vi "PE7265Monitor.vi"(0 "Lock-in Reference":u16(ring) items=["Lock-in 1", "Lock-in 2", "Lock-in 3"]) -> ()   [LabVIEW 2019]
uses:
  Utility/Monitor Communication/PE7265/PE7265-Cluster.ctl
  Utility/PE7260/PE7625-Settings.ctl
  Instrument_Setup.vi
  Global/Global Variables/Data_Display_global.vi
panel:
  out "PE7625-Settings":T1={"PE7265 AutoSens at ech step"=FALSE, "PE7265 Sens"=26, "Coupling"=FALSE, "AC Gain"=3, "Auto AC Gain"=FALSE, "Input Device (Voltage Mode)"=TRUE, "Line Frequency"=TRUE, "Input Connector Shells"=FALSE, "PE7265 Input Mode"=3, "Line Frequency\nRejection Filter"=1, "Port"=0, "7265 GPIB Address"=12, "Interface"=FALSE, "Exit"=FALSE, "GPIB Parameter 7260"={"address"="12", "delay time"=10.0, "mode"=6}, "PE7265 delay after AS"=10.0, "VISA session PE7265"="GPIB0::12::INSTR", "Slope"=1, "Synchronous TC"=TRUE, "Time Constant"=15, "Reference I/P"=0, "Reference\nHarmonic"=1, "Oscillator Amplitude (Volts rms)"=1.5, "Oscillator Frequency (Hz)"=19.0, "Ref Unlocked"=FALSE, "Virtual Reference\nMode"=FALSE} {"Oscillator Frequency (Hz)" min=0.001 max=250000.0 step=0.001 format="%.3f"; "Oscillator Amplitude (Volts rms)" min=0.0 max=5.0 step=1e-06 format="%.6f"; "Reference\nHarmonic" min=1 step=1; "Reference I/P" items=["Internal", "External TTL (Rear Panel)", "External (Front Panel)"]; "Time Constant" items=["10µs", "20µs", "40µs", "80µs", "160µs", "320µs", "640µs", "5ms", "10ms", "20ms", "50ms", "100ms", "200ms", "500ms", "1s", "2s", "5s", "10s", "20s", "50s", "100s", "200s", "500s", "1ks", "2ks", "5ks", "10ks", "20ks", "50ks", "100ks"]; "Slope" items=["6db/octave", "12dB/octave", "18dB/octave", "24dB/octave"]; "PE7265 delay after AS" format="%.2f"; "GPIB Parameter 7260"."delay time" format="%.2f"; "7265 GPIB Address" min=1 max=32 step=1; "Port" items=["COM 1", "COM 2", "COM 3", "COM 4", "COM 5", "COM 6", "COM 7", "COM 8", "COM 9", "COM 10"]; "Line Frequency\nRejection Filter" items=["OFF", "F", "2F", "F & 2F"]; "PE7265 Input Mode" items=["Inputs Grounded (test)", "A (Single-Ended Voltage)", "-B (Inverting Single Ended Voltage)", "A-B (Differential Voltage)", "B Current input - High Bandwidth", "B Current input - Low Noise"]; "AC Gain" items=["0dB", "10dB", "20dB", "30dB", "40dB", "50dB", "60dB", "70dB", "80dB", "90dB"]; "PE7265 Sens" items=["2nV", "5nV", "10nV", "20nV", "50nV", "100nV", "200nV", "500nV", "1µV", "2µV", "5µV", "10µV", "20µV", "50µV", "100µV", "200µV", "500µV", "1mV", "2mV", "5mV", "10mV", "20mV", "50mV", "100mV", "200mV", "500mV", "1V"]}
  out "Sensitivity 2":i16(ring)=15 items=["2 nV", "5 nV", "10 nV", "20 nV", "50 nV", "100 nV", "200 nV", "500 nV", "1 µV", "2 µV", "5 µV", "10 µV", "20 µV", "50 µV", "100 µV", "200 µV", "500 µV", "1 mV", "2 mV", "5 mV", "10 mV", "20 mV", "50 mV", "100 mV", "200 mV", "500 mV", "1 V", ""]
  in  "Stopp":bool
  out "PE7265-Cluster":T2={"Lockin 1"=[], "X1-Display"=0.0, "X1 Percent"=0.0, "Y1-Display"=0.0, "X1 Percent 2"=0.0, "Unit X1"="nV", "Unit X1a"="nV", "Unit X2"="nV", "Unit X2a"="nV", "X1 Overload"=FALSE, "Y1 Overload"=FALSE, "Sensitivity Setpoint"=26, "X1"=0.0, "Y1"=0.0} {"Sensitivity Setpoint" items=["2 nV", "5 nV", "10 nV", "20 nV", "50 nV", "100 nV", "200 nV", "500 nV", "1 µV", "2 µV", "5 µV", "10 µV", "20 µV", "50 µV", "100 µV", "200 µV", "500 µV", "1 mV", "2 mV", "5 mV", "10 mV", "20 mV", "50 mV", "100 mV", "200 mV", "500 mV", "1 V", ""]; "X1 Percent 2" scale=0.0..1.0; "X1 Percent" scale=0.0..1.0; "X1-Display" format="%#4_5f"}
  # "Input Configuration"
  # "RS232"
  # "GPIB"
  # "Uses VISA Communications"
  # "Sensitivity"
  # "Float"
  # "50 Hz"
  # "DC"
  # "Ground"
  # "60 Hz"
  # "AC"
  # "Bipolar - Input Impedance 10 k"
  # "On"
  # "FET - Input Impedance 10 M"
  # "Off"
  # "Output Channels"
  # "Reference Channel - Single Reference"
  # "On"
  # "Off"
  # "On"
  # "Off"
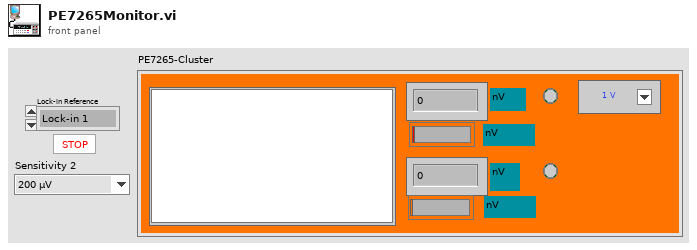
[diagram p1: front panel]
types:
  T1 = typedef "PE7625-Settings.ctl" = cluster{"PE7265 AutoSens at ech step":bool, "PE7265 Sens":i32, "Coupling":bool, "AC Gain":u16, "Auto AC Gain":bool, "Input Device (Voltage Mode)":bool, "Line Frequency":bool, "Input Connector Shells":bool, "PE7265 Input Mode":u16, "Line Frequency\nRejection Filter":u8, "Port":u16, "7265 GPIB Address":i8, "Interface":bool, "Exit":bool, "GPIB Parameter 7260":cluster{"address":string, "delay time":dbl, "mode":i32}, "PE7265 delay after AS":dbl, "VISA session PE7265":refnum<visa-resource-name>, "Slope":u8, "Synchronous TC":bool, "Time Constant":u16, "Reference I/P":u8, "Reference\nHarmonic":u16, "Oscillator Amplitude (Volts rms)":dbl, "Oscillator Frequency (Hz)":dbl, "Ref Unlocked":bool, "Virtual Reference\nMode":bool}
  T2 = typedef "PE7265-Cluster.ctl" = cluster{"Lockin 1":dbl[][], "X1-Display":dbl, "X1 Percent":dbl, "Y1-Display":dbl, "X1 Percent 2":dbl, "Unit X1":string, "Unit X1a":string, "Unit X2":string, "Unit X2a":string, "X1 Overload":bool, "Y1 Overload":bool, "Sensitivity Setpoint":i16, "X1":dbl, "Y1":dbl}
  T3 = cluster{"PE7265 AutoSens at ech step":bool, "PE7265 Sens":i32, "Coupling":bool, "AC Gain":u16, "Auto AC Gain":bool, "Input Device (Voltage Mode)":bool, "Line Frequency":bool, "Input Connector Shells":bool, "PE7265 Input Mode":u16, "Line Frequency\nRejection Filter":u8, "Port":u16, "7265 GPIB Address":i8, "Interface":bool, "Exit":bool, "GPIB Parameter 7260":cluster{"address":string, "delay time":dbl, "mode":i32}, "PE7265 delay after AS":dbl, "VISA session PE7265":refnum<visa-resource-name>, "Slope":u8, "Synchronous TC":bool, "Time Constant":u16, "Reference I/P":u8, "Reference\nHarmonic":u16, "Oscillator Amplitude (Volts rms)":dbl, "Oscillator Frequency (Hz)":dbl, "Ref Unlocked":bool, "Virtual Reference\nMode":bool}
  T4 = cluster{"address":string, "delay time":dbl, "mode":i32}
  T5 = cluster{"Sensitivity Setpoint 1":i32, "Sensitivity Setpoint 2":i32, "Sensitivity Setpoint 3":i32}
  T6 = cluster{"LIA7230-Running":bool, "LIA7230-Running 2":bool, "LIA7230-Running 3":bool, "SR830-Running":bool, "SR830-Running 2":bool, "SR830-Running 3":bool, "PE7265-running":bool, "zurich_Lock_in-running":bool}
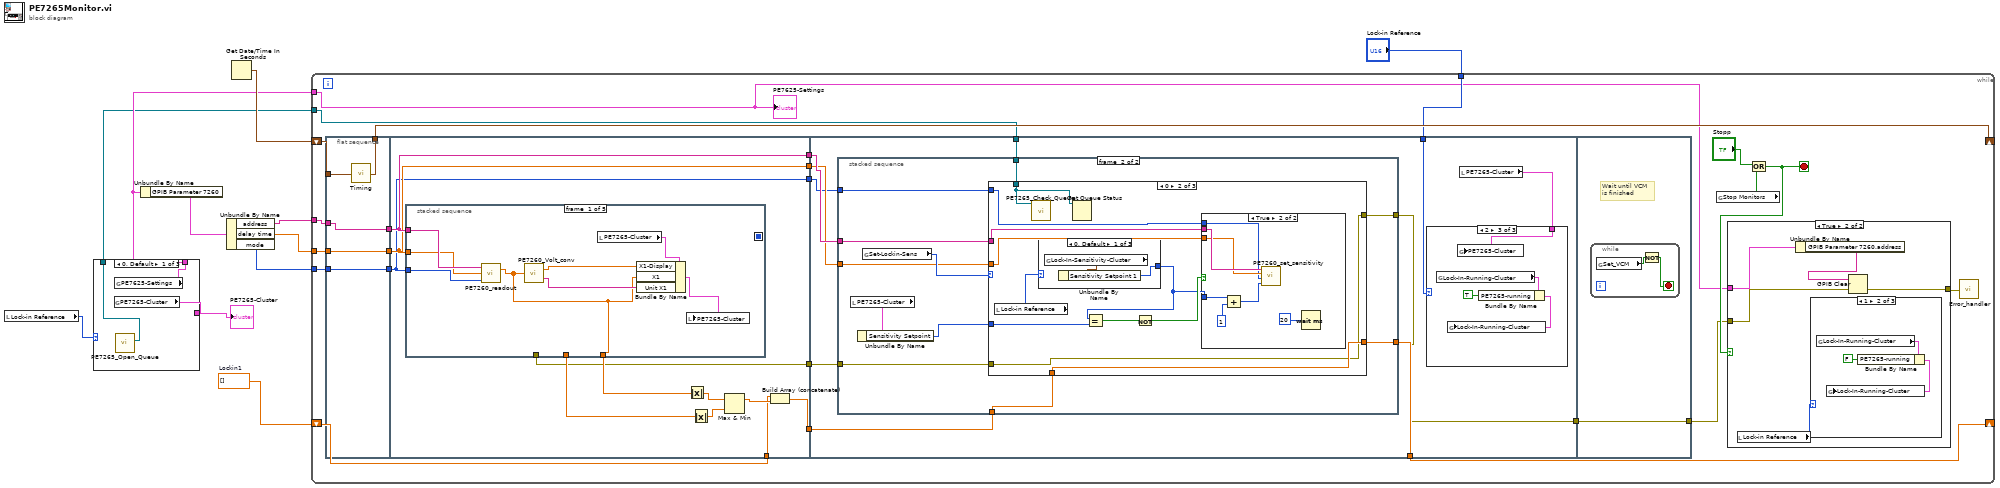
[diagram p0: block diagram]
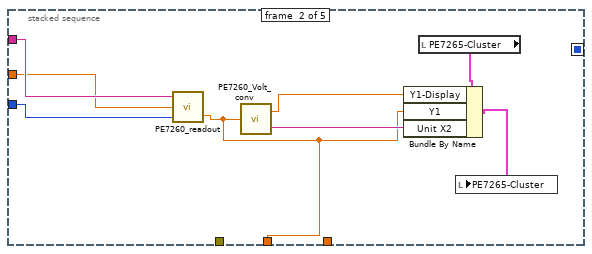
[diagram p2: hidden frame]
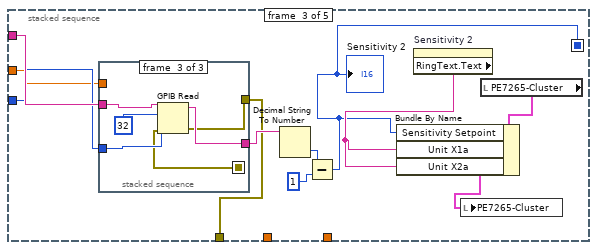
[diagram p3: hidden frame]
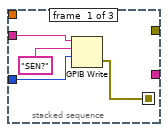
[diagram p4: hidden frame]
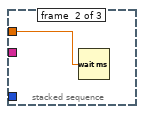
[diagram p5: hidden frame]
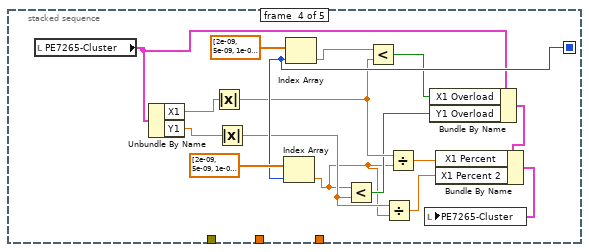
[diagram p6: hidden frame]
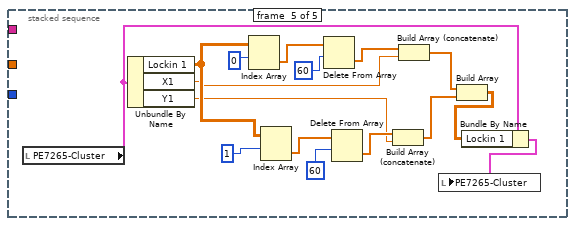
[diagram p7: hidden frame]
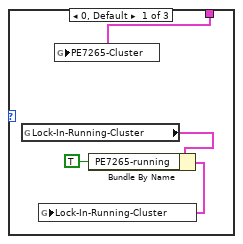
[diagram p8: hidden frame]
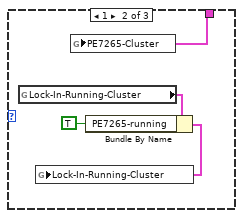
[diagram p9: hidden frame]
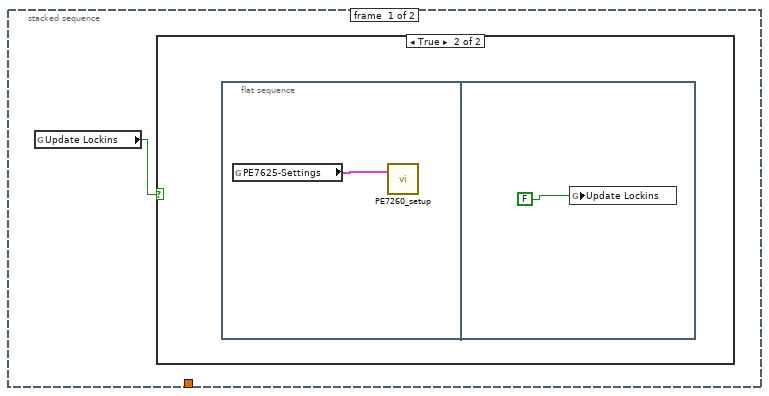
[diagram p10: hidden frame]
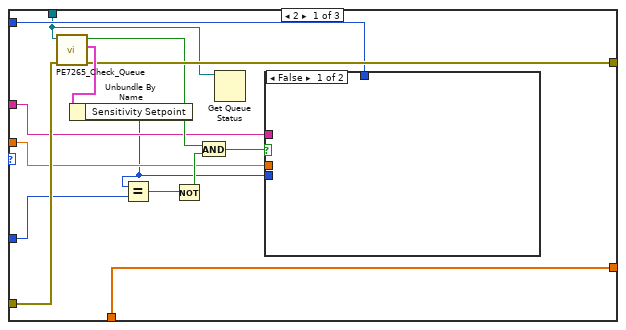
[diagram p12: hidden frame]
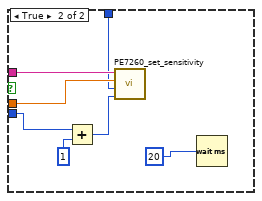
[diagram p13: hidden frame]
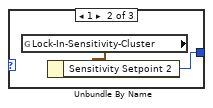
[diagram p15: hidden frame]
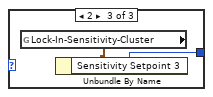
[diagram p16: hidden frame]
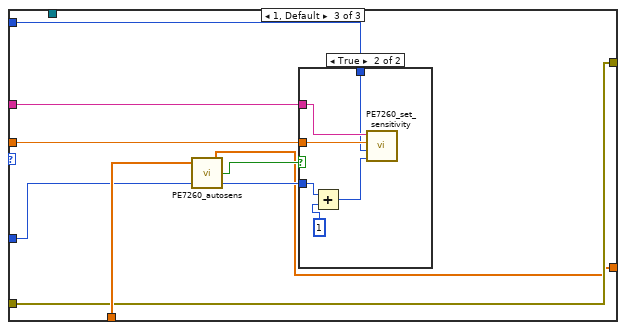
[diagram p17: hidden frame]
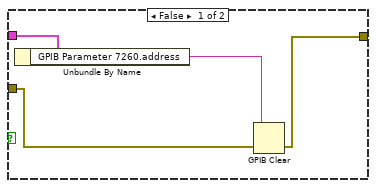
[diagram p19: hidden frame]
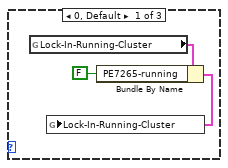
[diagram p20: hidden frame]
diagram:
  w4 = dbl[] []  # Lockin1
  n1 = local read "Lock-in Reference"() -> (w11:u16)
  n2 = case shown="0, Default" w11 {
    tunnel: [w14 w17 w20] -> w7
    tunnel: [w13 w16 w19] -> w10
    tunnel: [w12 w15 w18] -> w3
    frame 0, Default {
      n3 = global read "Data_Display_global.vi" "PE7265-Cluster"() -> (w13:T2)
      n4 = global read "Instrument_Setup.vi" "PE7625-Settings"() -> (w14:T3)
      n5 = call "PE7265_Open_Queue.vi"() -> ("queue out"=w12:refnum<queue>)  [unwired: 10 in, 1 out]
    }
    frame 2 {
      n6 = global read "Instrument_Setup.vi" "PE7625-Settings"() -> (w17:T3)
      n7 = global read "Data_Display_global.vi" "PE7265-Cluster"() -> (w16:T2)
      n8 = call "PE7265_Open_Queue.vi"() -> ("queue out"=w15:refnum<queue>)  [unwired: 10 in, 1 out]
    }
    frame 1 {
      n9 = global read "Instrument_Setup.vi" "PE7625-Settings"() -> (w20:T3)
      n10 = global read "Data_Display_global.vi" "PE7265-Cluster"() -> (w19:T2)
      n11 = call "PE7265_Open_Queue.vi"() -> ("queue out"=w18:refnum<queue>)  [unwired: 10 in, 1 out]
    }
  }
  "PE7265-Cluster" <- w10
  n12 = Unbundle By Name(w7) -> ("GPIB Parameter 7260"=w9:T4)
  n13 = Unbundle By Name(w9) -> ("address"=w1:string, "delay time"=w6:dbl, "mode"=w5:i32)
  n14 = Get Date/Time In Seconds() -> (seconds since 1Jan1904=w8:timestamp)
  n15 = while {
    tunnel: w1 -> [w39]
    shift-right: [w40] -> _
    shift-left: w8 -> [w41]
    tunnel: w7 -> [w21]
    tunnel: w6 -> [w37]
    tunnel: w5 -> [w35]
    shift-right: [w25] -> _
    shift-left: w4 -> [w33]
    tunnel: w3 -> [w24]
    tunnel: "Lock-in Reference" -> [w23]
    stop <- w27 stop-if-true
    n16 = flat-sequence {
      tunnel: w41 -> [w49]
      tunnel: [w48] -> w40
      tunnel: w39 -> [w47]
      tunnel: [w47] -> w38
      tunnel: w37 -> [w46]
      tunnel: [w46] -> w36
      tunnel: w35 -> [w45]
      tunnel: [w45] -> w34
      tunnel: w38 -> [w52]
      tunnel: w36 -> [w51]
      tunnel: w34 -> [w50]
      tunnel: w33 -> [w57]
      tunnel: [w54] -> w32
      tunnel: [w53] -> w31
      tunnel: [w52] -> w30
      tunnel: [w51] -> w29
      tunnel: [w50] -> w28
      tunnel: w32 -> [w140]
      tunnel: w31 -> [w135]
      tunnel: w30 -> [w139]
      tunnel: w29 -> [w138]
      tunnel: w28 -> [w137]
      tunnel: [w136] -> w25
      tunnel: w24 -> [w133]
      tunnel: w23 -> [w132]
      tunnel: [w134] -> w22
      tunnel: [w227] -> w26
      tunnel: w22 -> [w227]
      frame #0 {
        n17 = call "Timing.vi"("start time (s)"=w49) -> ("last reading (s)"=w48:timestamp)
      }
      frame #1 {
        n18 = stacked-sequence {
          seq-local: [_ _ w77 _ _] -> [_ _ _ w112 _]
          tunnel: w52 -> [w67 w76 w87 _ _]
          tunnel: w51 -> [w66 w75 w85 _ _]
          tunnel: w50 -> [w65 w74 w86 _ _]
          tunnel: [w62 _ _ _ _] -> w60
          tunnel: [_ w69 _ _ _] -> w56
          tunnel: [_ _ w81 _ _] -> w53
          frame #0 {
            n19 = call "PE7260_readout.vi"("mode"=w65, "delay time"=w66, "address"=w67) -> ("7265 X"=w62:dbl)  [unwired: 1 out]
            n20 = call "PE7260_Volt_conv.vi"("Numerisch"=w62) -> ("Numerisch 2"=w64:dbl, "String"=w63:string)
            n21 = local read "PE7265-Cluster"() -> (w68:T2)
            n22 = Bundle By Name(cluster=w68, "X1-Display"=w64, "X1"=w62, "Unit X1"=w63) -> (w61:T2)
            n23 = local write "PE7265-Cluster"(w61) -> ()
          }
          frame #1 {
            n24 = call "PE7260_readout.vi"("mode"=w74, "delay time"=w75, "address"=w76) -> ("7265 Y"=w69:dbl)  [unwired: 1 out]
            n25 = call "PE7260_Volt_conv.vi"("Numerisch"=w69) -> ("Numerisch 2"=w71:dbl, "String"=w70:string)
            n26 = local read "PE7265-Cluster"() -> (w73:T2)
            n27 = Bundle By Name(cluster=w73, "Y1-Display"=w71, "Y1"=w69, "Unit X2"=w70) -> (w72:T2)
            n28 = local write "PE7265-Cluster"(w72) -> ()
          }
          frame #2 {
            n29 = stacked-sequence {
              seq-local: [w88 _ _] -> [_ _ w94]
              tunnel: w87 -> [w91 _ w96]
              tunnel: w86 -> [w90 _ w97]
              tunnel: w85 -> [_ w92 _]
              tunnel: [_ _ w95] -> w84
              tunnel: [_ _ w93] -> w81
              frame #0 {
                n30 = GPIB Write(0:w91, 1:"SEN?", 2:w90) -> (6:w88:errorcluster)  [unwired: 2 in, 1 out]
              }
              frame #1 {
                n31 = Wait (ms)(milliseconds to wait=w92) -> ()  [unwired: 1 out]
              }
              frame #2 {
                n32 = GPIB Read(0:w96, 1:32, 2:w97, 3:w94) -> (5:w95:string, 7:w93:errorcluster)  [unwired: 1 in, 1 out]
              }
            }
            n33 = Decimal String To Number(string=w84) -> (number=w79:i32)  [unwired: 2 in, 1 out]
            n34 = Subtract(x=w79, y=1) -> (x-y=w77:i32)
            "Sensitivity 2" <- w77
            n35 = property on="Sensitivity 2" class="Ring (strict)"() -> ("RingText.Text"=w80:string)  [unwired: 2 in, 2 out]
            n36 = local read "PE7265-Cluster"() -> (w83:T2)
            n37 = Bundle By Name(cluster=w83, "Sensitivity Setpoint"=w77, "Unit X1a"=w80, "Unit X2a"=w80) -> (w82:T2)
            n38 = local write "PE7265-Cluster"(w82) -> ()
          }
          frame #3 {
            n39 = local read "PE7265-Cluster"() -> (w108:T2)
            n40 = Unbundle By Name(w108) -> ("X1"=w111:dbl, "Y1"=w110:dbl)
            n41 = Absolute Value(x=w111) -> (abs(x)=w104:dbl)
            n42 = Absolute Value(x=w110) -> (abs(x)=w101:dbl)
            n43 = Index Array(array=dbl[] [2e-09, 5e-09, 1e-08, 2e-08, 5e-08, 1e-07, 2e-07, 5e-07, 1e-06, 2e-06, 5e-06, 1e-05, 2e-05, 5e-05, 0.0001, 0.0002, 0.0005, 0.001, 0.002, 0.005, 0.01, 0.02, 0.05, 0.1, 0.2, 0.5, 1.0] ("Array"), index=w112) -> (element=w100:dbl)
            n44 = Index Array(array=dbl[] [2e-09, 5e-09, 1e-08, 2e-08, 5e-08, 1e-07, 2e-07, 5e-07, 1e-06, 2e-06, 5e-06, 1e-05, 2e-05, 5e-05, 0.0001, 0.0002, 0.0005, 0.001, 0.002, 0.005, 0.01, 0.02, 0.05, 0.1, 0.2, 0.5, 1.0] ("Array"), index=w112) -> (element=w109:dbl)
            n45 = Less?(x=w100, y=w101) -> (x < y?=w102:bool)
            n46 = Less?(x=w109, y=w104) -> (x < y?=w105:bool)
            n47 = Divide(x=w101, y=w100) -> (x/y=w99:dbl)
            n48 = Divide(x=w104, y=w100) -> (x/y=w103:dbl)
            n49 = Bundle By Name(cluster=w108, "X1 Overload"=w105, "Y1 Overload"=w102) -> (w107:T2)
            n50 = Bundle By Name(cluster=w107, "X1 Percent"=w103, "X1 Percent 2"=w99) -> (w106:T2)
            n51 = local write "PE7265-Cluster"(w106) -> ()
          }
          frame #4 {
            n52 = local read "PE7265-Cluster"() -> (w117:T2)
            n53 = Unbundle By Name(w117) -> ("Lockin 1"=w129:dbl[][], "X1"=w124:dbl, "Y1"=w120:dbl)
            n54 = Index Array(array=w129, index (row)=0) -> (element=w127:dbl[])  [unwired: 1 in]
            n55 = Index Array(array=w129, index (row)=1) -> (element=w123:dbl[])  [unwired: 1 in]
            n56 = Delete From Array(array=w127, length=60) -> (deleted portion=w125:dbl[])  [unwired: 1 in, 1 out]
            n57 = Delete From Array(array=w123, length=60) -> (deleted portion=w121:dbl[])  [unwired: 1 in, 1 out]
            n58 = Build Array (concatenate)(w121, w120) -> (w118:dbl[])
            n59 = Build Array (concatenate)(w125, w124) -> (w119:dbl[])
            n60 = Build Array(w119, w118) -> (w116:dbl[][])
            n61 = Bundle By Name(cluster=w117, "Lockin 1"=w116) -> (w115:T2)
            n62 = local write "PE7265-Cluster"(w115) -> ()
          }
        }
        n63 = Absolute Value(x=w60) -> (abs(x)=w59:dbl)
        n64 = Absolute Value(x=w56) -> (abs(x)=w55:dbl)
        n65 = Max & Min(x=w59, y=w55) -> (max(x,y)=w58:dbl)  [unwired: 1 out]
        n66 = Build Array (concatenate)(w57, w58) -> (w54:dbl[])
      }
      frame #2 {
        n67 = stacked-sequence {
          tunnel: w140 -> [_ w163]
          tunnel: w139 -> [_ w162]
          tunnel: w138 -> [_ w161]
          tunnel: w137 -> [_ w160]
          tunnel: [_ w156] -> w136
          tunnel: w135 -> [_ w159]
          tunnel: [_ w158] -> w134
          tunnel: w133 -> [_ w157]
          frame #0 {
            n68 = global read "Instrument_Setup.vi" "Update Lockins"() -> (w153:bool)
            n69 = case shown="True" w153 {
              frame False {
              }
              frame True {
                n70 = flat-sequence {
                  frame #0 {
                    n71 = global read "Instrument_Setup.vi" "PE7625-Settings"() -> (w154:T3)
                    n72 = call "PE7260_setup.vi"("PE7625-Settings"=w154) -> ()  [unwired: 2 in]
                  }
                  frame #1 {
                    n73 = global write "Instrument_Setup.vi" "Update Lockins"(FALSE) -> ()
                  }
                }
              }
            }
          }
          frame #1 {
            n74 = local read "PE7265-Cluster"() -> (w165:T2)
            n75 = Unbundle By Name(w165) -> ("Sensitivity Setpoint"=w164:i16)
            n76 = global read "Instrument_Setup.vi" "Set-Lockin-Sens"() -> (w166:u16)
            n77 = case shown="0" w166 {
              tunnel: w164 -> [w177 w196 w219]
              tunnel: w163 -> [w167 w189 w220]
              tunnel: w162 -> [w172 w193 w217]
              tunnel: w161 -> [w171 w192 w216]
              tunnel: w160 -> [w170 w191 w215]
              tunnel: w159 -> [w180 w188 w213]
              tunnel: [w178 w188 w213] -> w158
              tunnel: w157 -> [w168 w198 _]
              tunnel: [w167 w189 w212] -> w156
              frame 2 {
                n78 = call "PE7265_Check_Queue.vi"("error in (no error)"=w180, "queue"=w168) -> ("error out"=w178:errorcluster, "PE7265-Cluster"=w179:T2, "New Entries?"=w175:bool)  [unwired: 6 in]
                n79 = Unbundle By Name(w179) -> ("Sensitivity Setpoint"=w169:i16)
                n80 = Equal?(x=w169, y=w177) -> (x = y?=w176:bool)
                n81 = Not(x=w176) -> (.not. x?=w174:bool)
                n82 = And(x=w175, y=w174) -> (x .and. y?=w173:bool)
                n83 = Get Queue Status(queue=w168) -> ()  [unwired: 2 in, 8 out]
                n84 = case shown="False" w173 {
                  tunnel: w172 -> [_ w187]
                  tunnel: w171 -> [_ w186]
                  tunnel: w170 -> [_ w185]
                  tunnel: w169 -> [_ w183]
                  frame False {
                  }
                  frame True {
                    n85 = Add(x=w183, y=1) -> (x+y=w181:i32)
                    n86 = call "PE7260_set_sensitivity.vi"("Address"=w187, "delay time"=w186, "mode"=w185, "SEN 7265"=w181) -> ()  [unwired: 6 in]
                    n87 = Wait (ms)(milliseconds to wait=20) -> ()  [unwired: 1 out]
                  }
                }
              }
              frame 0 {
                n88 = local read "Lock-in Reference"() -> (w197:u16)
                n89 = call "PE7265_Check_Queue.vi"("queue"=w198) -> ()  [unwired: 7 in, 3 out]
                n90 = case shown="0, Default" w197 {
                  tunnel: [w206 w208 w210] -> w190
                  frame 0, Default {
                    n91 = global read "Data_Display_global.vi" "Lock-In-Sensitivity-Cluster"() -> (w207:T5)
                    n92 = Unbundle By Name(w207) -> ("Sensitivity Setpoint 1"=w206:i32)
                  }
                  frame 1 {
                    n93 = global read "Data_Display_global.vi" "Lock-In-Sensitivity-Cluster"() -> (w209:T5)
                    n94 = Unbundle By Name(w209) -> ("Sensitivity Setpoint 2"=w208:i32)
                  }
                  frame 2 {
                    n95 = global read "Data_Display_global.vi" "Lock-In-Sensitivity-Cluster"() -> (w211:T5)
                    n96 = Unbundle By Name(w211) -> ("Sensitivity Setpoint 3"=w210:i32)
                  }
                }
                n97 = Get Queue Status(queue=w198) -> ()  [unwired: 2 in, 8 out]
                n98 = Equal?(x=w190, y=w196) -> (x = y?=w195:bool)
                n99 = Not(x=w195) -> (.not. x?=w194:bool)
                n100 = case shown="True" w194 {
                  tunnel: w193 -> [_ w205]
                  tunnel: w192 -> [_ w204]
                  tunnel: w191 -> [_ w203]
                  tunnel: w190 -> [_ w201]
                  frame False {
                  }
                  frame True {
                    n101 = Add(x=w201, y=1) -> (x+y=w199:i32)
                    n102 = call "PE7260_set_sensitivity.vi"("Address"=w205, "delay time"=w204, "mode"=w203, "SEN 7265"=w199) -> ()  [unwired: 6 in]
                    n103 = Wait (ms)(milliseconds to wait=20) -> ()  [unwired: 1 out]
                  }
                }
              }
              frame 1, Default {
                n104 = call "PE7260_autosens.vi"("Sensitivity"=w219, "Data in"=w220) -> ("Sensitivity Out"=w214:i32, "Set Sensitivity"=w218:bool, "Data out"=w212:dbl[])  [unwired: 1 in]
                n105 = case shown="True" w218 {
                  tunnel: w217 -> [_ w226]
                  tunnel: w216 -> [_ w225]
                  tunnel: w215 -> [_ w224]
                  tunnel: w214 -> [_ w223]
                  frame False {
                  }
                  frame True {
                    n106 = Add(x=w223, y=1) -> (x+y=w221:i32)
                    n107 = call "PE7260_set_sensitivity.vi"("Address"=w226, "delay time"=w225, "mode"=w224, "SEN 7265"=w221) -> ()  [unwired: 6 in]
                  }
                }
              }
            }
          }
        }
        n108 = local read "PE7265-Cluster"() -> (w131:T2)
        n109 = case shown="2" w132 {
          tunnel: w131 -> [w144 w148 w152]
          frame 0, Default {
            n110 = global read "Data_Display_global.vi" "Lock-In-Running-Cluster"() -> (w143:T6)
            n111 = global write "Data_Display_global.vi" "PE7265-Cluster"(w144) -> ()
            n112 = Bundle By Name(cluster=w143, "PE7265-running"=TRUE) -> (w141:T6)
            n113 = global write "Data_Display_global.vi" "Lock-In-Running-Cluster"(w141) -> ()
          }
          frame 1 {
            n114 = global read "Data_Display_global.vi" "Lock-In-Running-Cluster"() -> (w145:T6)
            n115 = global write "Data_Display_global.vi" "PE7265-Cluster"(w148) -> ()
            n116 = Bundle By Name(cluster=w145, "PE7265-running"=TRUE) -> (w146:T6)
            n117 = global write "Data_Display_global.vi" "Lock-In-Running-Cluster"(w146) -> ()
          }
          frame 2 {
            n118 = global read "Data_Display_global.vi" "Lock-In-Running-Cluster"() -> (w149:T6)
            n119 = global write "Data_Display_global.vi" "PE7265-Cluster"(w152) -> ()
            n120 = Bundle By Name(cluster=w149, "PE7265-running"=TRUE) -> (w150:T6)
            n121 = global write "Data_Display_global.vi" "Lock-In-Running-Cluster"(w150) -> ()
          }
        }
      }
      frame #3 {
        # "Wait until VCM \nis finished"
        n122 = while {
          stop <- w228 stop-if-true
          n123 = global read "Data_Display_global.vi" "Set_VCM"() -> (w229:bool)
          n124 = Not(x=w229) -> (.not. x?=w228:bool)
        }
      }
    }
    n125 = global read "Data_Display_global.vi" "Stop Monitors"() -> (w43:bool)
    n126 = Or(x="Stopp", y=w43) -> (x .or. y?=w27:bool)
    n127 = case shown="True" w27 {
      tunnel: [w230 w234] -> w42
      tunnel: w26 -> [w231 w238]
      tunnel: w21 -> [w233 w237]
      frame False {
        n128 = Unbundle By Name(w233) -> ("GPIB Parameter 7260.address"=w232:string)
        n129 = GPIB Clear(2:w231, 3:w232) -> (0:w230:errorcluster)  [unwired: 1 out]
      }
      frame True {
        n130 = local read "Lock-in Reference"() -> (w236:u16)
        n131 = Unbundle By Name(w237) -> ("GPIB Parameter 7260.address"=w235:string)
        n132 = case shown="1" w236 {
          frame 0, Default {
            n133 = global read "Data_Display_global.vi" "Lock-In-Running-Cluster"() -> (w239:T6)
            n134 = Bundle By Name(cluster=w239, "PE7265-running"=FALSE) -> (w240:T6)
            n135 = global write "Data_Display_global.vi" "Lock-In-Running-Cluster"(w240) -> ()
          }
          frame 1 {
            n136 = global read "Data_Display_global.vi" "Lock-In-Running-Cluster"() -> (w242:T6)
            n137 = Bundle By Name(cluster=w242, "PE7265-running"=FALSE) -> (w243:T6)
            n138 = global write "Data_Display_global.vi" "Lock-In-Running-Cluster"(w243) -> ()
          }
          frame 2 {
            n139 = global read "Data_Display_global.vi" "Lock-In-Running-Cluster"() -> (w245:T6)
            n140 = Bundle By Name(cluster=w245, "PE7265-running"=FALSE) -> (w246:T6)
            n141 = global write "Data_Display_global.vi" "Lock-In-Running-Cluster"(w246) -> ()
          }
        }
        n142 = GPIB Clear(2:w238, 3:w235) -> (0:w234:errorcluster)  [unwired: 1 out]
      }
    }
    n143 = call "Error_handler.vi"("error constant"=w42) -> ()
    "PE7625-Settings" <- w21
  }
